vi "PositionReceiverAngleAttacker.vi"(6 "AnguloGol":dbl, 8 "error in (no error)":errorcluster, 9 "atacando contra":bool, 10 "Game":refnum<class "Game.lvclass">, 11 "PositionToReceivePassSkill in":refnum<class "PositionToReceivePassSkill.lvclass">) -> (0 "error out":errorcluster, 1 "AttackerPositive?":bool, 2 "theta final":dbl, 3 "PositionToReceivePassSkill out":refnum<class "PositionToReceivePassSkill.lvclass">, 4 "YdoAttacker 2":dbl, 5 "XdoAttacker 2":dbl)   [LabVIEW 2023, in "PositionToReceivePassSkill.lvclass"]
uses:
  PositionToReceivePassSkill.lvclass
  Game_class/Game.lvclass
  Game_class/Game.lvclass/Game.ctl
  Team_class/Team.lvclass/Team.ctl
  Object_class/Object.lvclass/Object.ctl
  Robot_class/Robot.lvclass/Robot.ctl
  Object_class/Read x.vi
  Object_class/Write x.vi
  Object_class/Read y.vi
  Robot_class/Read id.vi
  Game_class/Read OffensiveTeam.vi
  Game_class/Read EnemyRef.vi
  Game_class/Read FieldRef.vi
  Game_class/Read DefensiveTeam.vi
  Game_class/Read KeeperTeam.vi
  Game_class/Read BallRef.vi
  Team_class/Read RobotRef.vi
  Ball_class/Ball.lvclass
  Ally_class/Ally.lvclass
  Enemy_class/Enemy.lvclass
  Robot_class/Robot.lvclass
  Field_class/Field.lvclass
panel:
  in  "valor de theta 3":dbl
  in  "tamanho do intervalo 3":dbl
  in  "inicio do intervalo 3":dbl
  in  "fim do intervalo 3":dbl
  in  "Contador 4":dbl
  in  "Array 3":dbl[](array[numeric])=[0.0, 0.0, 0.0, 0.0, 0.0, 0.0]
  in  "valor de theta 2":dbl
  in  "tamanho do intervalo 2":dbl
  in  "inicio do intervalo 2":dbl
  in  "fim do intervalo 2":dbl
  in  "Contador 3":dbl
  in  "Array 2":dbl[](array[numeric])=[0.0, 0.0, 0.0, 0.0, 0.0, 0.0]
  in  "RobôsParaAnalisar":dbl[][](array[numeric])=[[99999.0, 99999.0], [99999.0, 99999.0], [99999.0, 99999.0], [99999.0, 99999.0], [99999.0, 99999.0], [99999.0, 99999.0], [99999.0, 99999.0]]
  in  "Contador":dbl
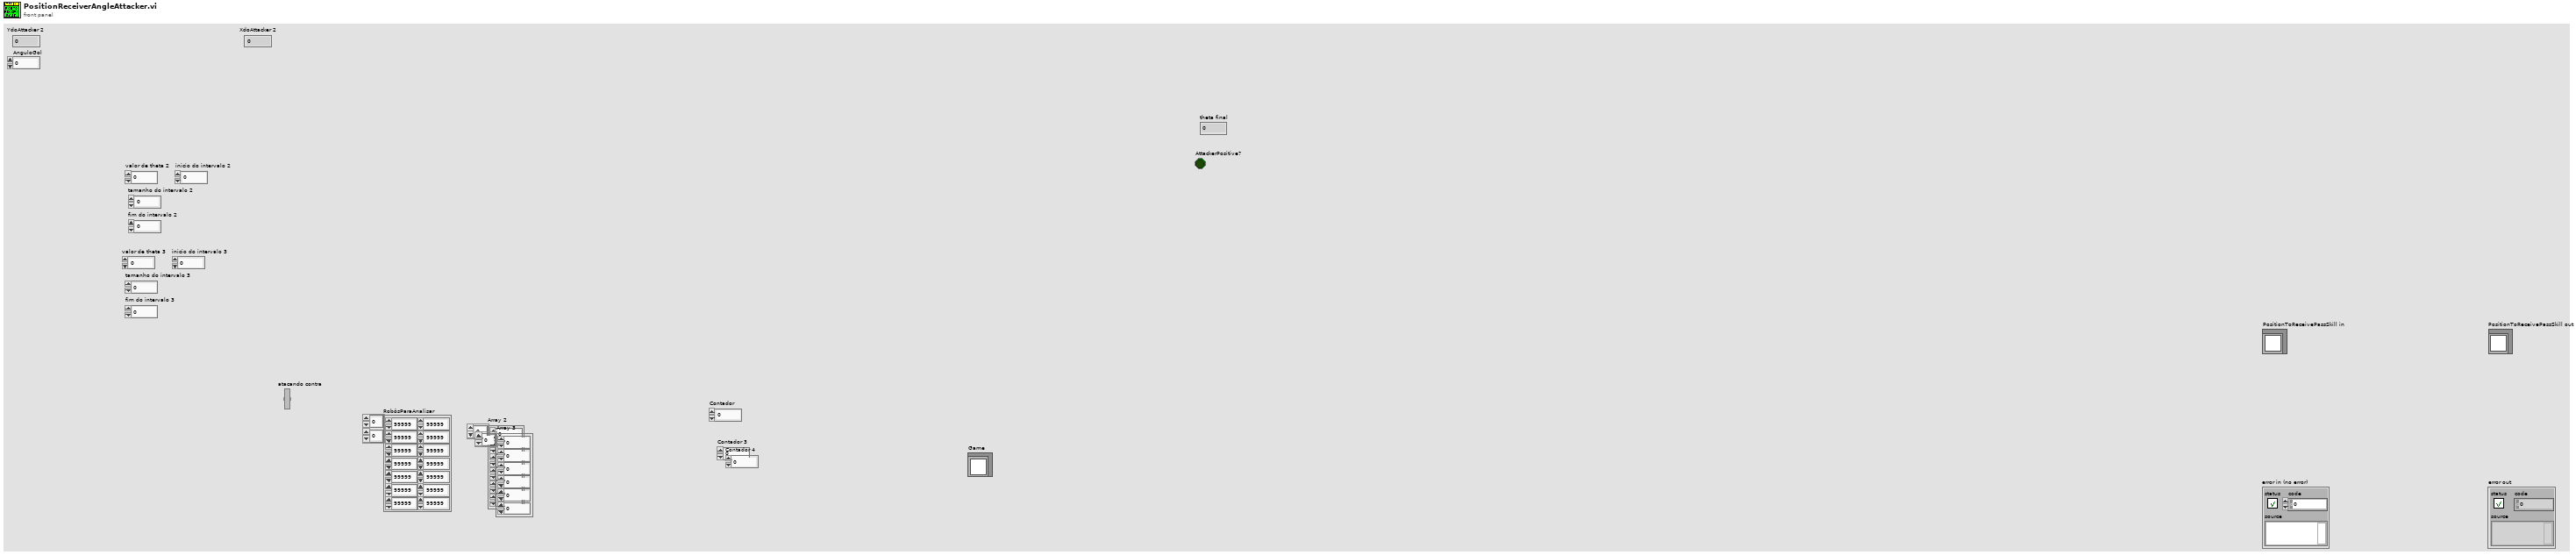
[diagram p1: front panel]
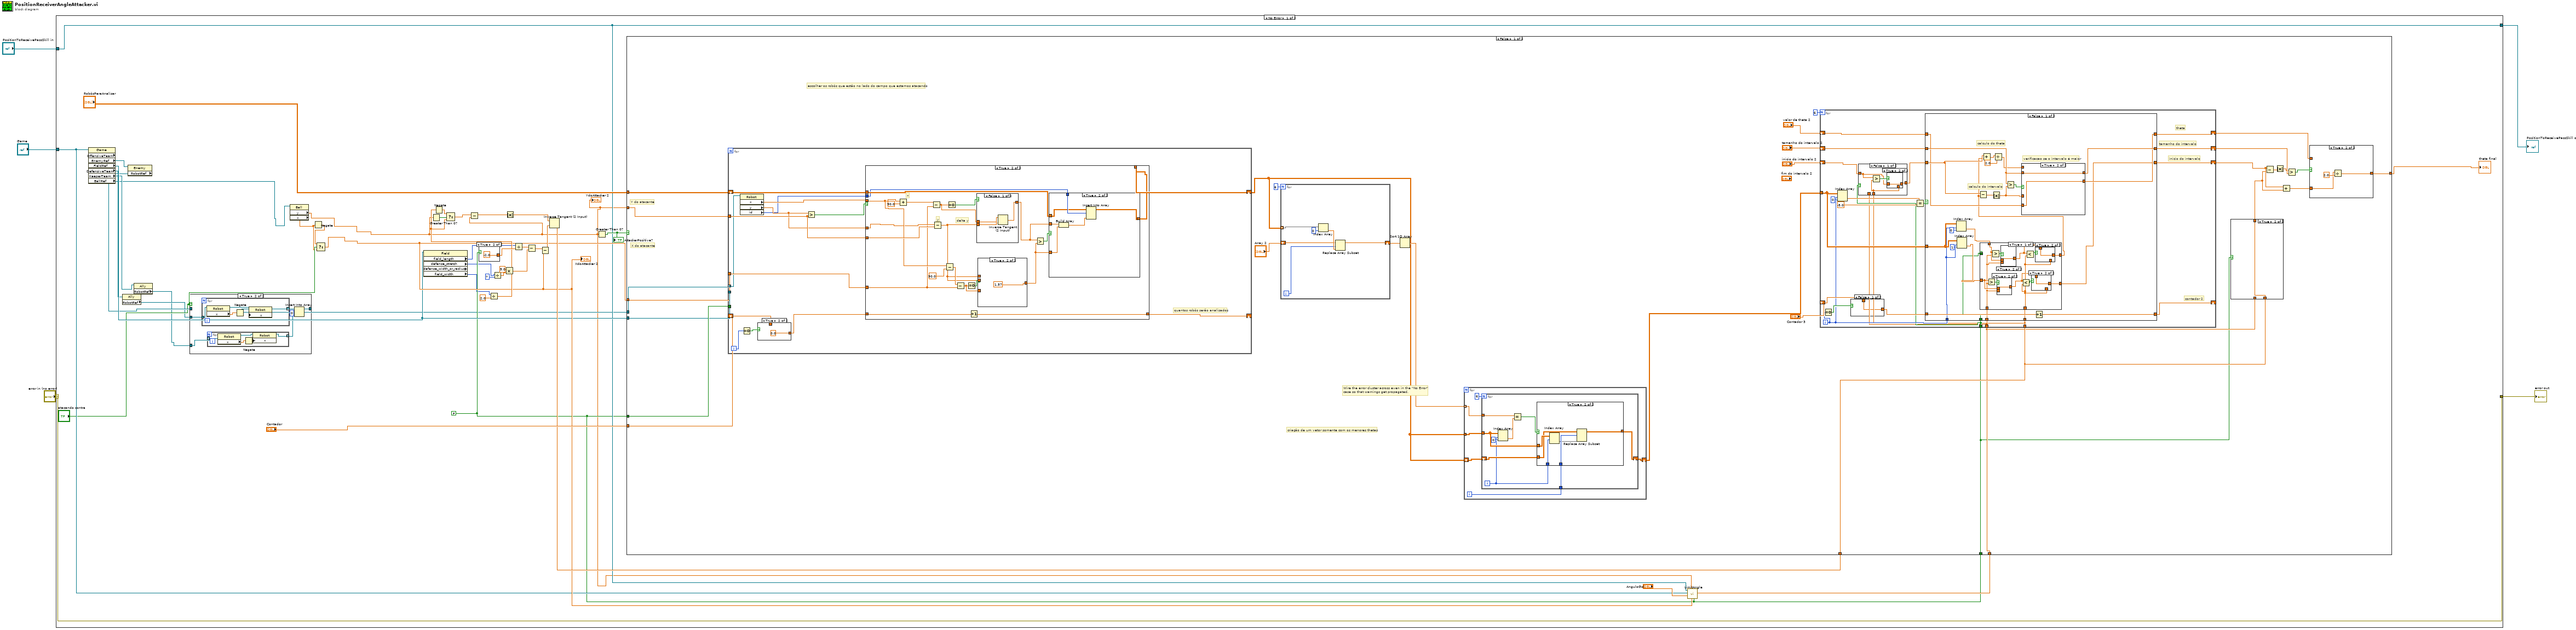
[diagram p0: block diagram]
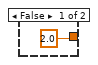
[diagram p3: hidden frame]
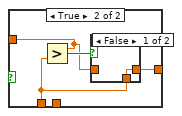
[diagram p8: hidden frame]
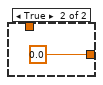
[diagram p10: hidden frame]
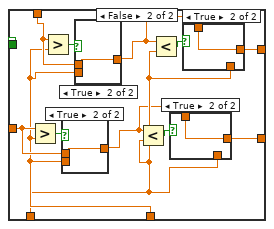
[diagram p15: hidden frame]
diagram:
  n1 = case shown="No Error" "error in (no error)" {
    selector: "error in (no error)" -> [w48 w537]
    tunnel: [w48 w537] -> w4
    tunnel: [w25 w536] -> w2
    tunnel: "PositionToReceivePassSkill in" -> [w25 w536]
    tunnel: "Game" -> [w26 _]
    frame No Error {
      w20 = FALSE ("atacando contra")
      # "Wire the error cluster across even in the \"No Error\"\ncase so that warnings get propagated."
      n2 = property class="Game" props=["OffensiveTeam", "EnemyRef", "FieldRef", "DefensiveTeam", "KeeperTeam", "BallRef"](reference=w26) -> ("EnemyRef"=w29:refnum<class "Enemy.lvclass">, "FieldRef"=w28:refnum<class "Field.lvclass">, "DefensiveTeam"=w15:refnum<class "Ally.lvclass">, "KeeperTeam"=w13:refnum<class "Ally.lvclass">, "BallRef"=w11:refnum<class "Ball.lvclass">)  [unwired: 1 in, 3 out]
      n3 = property class="Ally"(reference=w15) -> ("RobotRef"=w14:refnum<class "Robot.lvclass">[])  [unwired: 1 in, 2 out]
      n4 = property class="Enemy"(reference=w29) -> ("RobotRef"=w18:refnum<class "Robot.lvclass">[])  [unwired: 1 in, 2 out]
      n5 = property class="Ally"(reference=w13) -> ("RobotRef"=w12:refnum<class "Robot.lvclass">[])  [unwired: 1 in, 2 out]
      n6 = case shown="True" "atacando contra" {
        tunnel: [w49 w50] -> w19
        tunnel: w18 -> [w49 _]
        tunnel: w14 -> [_ w55]
        tunnel: w12 -> [_ w54]
        frame False {
        }
        frame True {
          n7 = for {
            tunnel: [w63] -> w53 mode=indexing
            tunnel: w55 -> [w61] mode=indexing
            n8 = property class="Robot"(reference=w61) -> (reference out=w62:refnum<class "Robot.lvclass">, "x"=w65:dbl)  [unwired: 1 in, 1 out]
            n9 = Negate(x=w65) -> (-x=w64:dbl)
            n10 = property class="Robot"(reference=w62, "x"=w64) -> (reference out=w63:refnum<class "Robot.lvclass">)  [unwired: 1 in, 1 out]
          }
          n11 = for {
            tunnel: w54 -> [w60] mode=indexing
            tunnel: [w56] -> w52 mode=indexing
            n12 = property class="Robot"(reference=w60) -> (reference out=w57:refnum<class "Robot.lvclass">, "x"=w59:dbl)  [unwired: 1 in, 1 out]
            n13 = Negate(x=w59) -> (-x=w58:dbl)
            n14 = property class="Robot"(reference=w57, "x"=w58) -> (reference out=w56:refnum<class "Robot.lvclass">)  [unwired: 1 in, 1 out]
          }
          n15 = Insert Into Array(array=w53, index=0, new element=w52) -> (w50:refnum<class "Robot.lvclass">[])
        }
      }
      n16 = property class="Ball"(reference=w11) -> ("y"=w9:dbl, "x"=w8:dbl)  [unwired: 1 in, 2 out]
      "YdoAttacker 2" <- w9
      n17 = Negate(x=w8) -> (-x=w10:dbl)
      n18 = Select(t=w10, s="atacando contra", f=w8) -> (s? t:f=w34:dbl)
      "XdoAttacker 2" <- w34
      n19 = property class="Field" props=["field_length", "defense_stretch", "defense_width_or_radius", "field_width"](reference=w28) -> ("field_length"=w27:i32, "defense_stretch"=w7:i32, "field_width"=w6:i32)  [unwired: 1 in, 3 out]
      n20 = Greater Than 0?(x=w9) -> (x > 0?=w44:bool)
      n21 = case shown="True" w20 {
        tunnel: [2.0 ("y") -2.0 ("y")] -> w42
        frame False {
        }
        frame True {
        }
      }
      n22 = Divide(x=w6, y=2.0) -> (x/y=w40:dbl)
      n23 = Negate(x=w40) -> (-x=w43:dbl)
      n24 = Select(t=w43, s=w44, f=w40) -> (s? t:f=w36:dbl)
      n25 = Subtract(x=w36, y=w9) -> (x-y=w33:dbl)
      n26 = Divide(x=w7, y=7) -> (x/y=w23:dbl)
      n27 = Multiply(x=5.0, y=w23) -> (x*y=w21:dbl)
      n28 = Absolute Value(x=w33) -> (abs(x)=w32:dbl)
      n29 = Divide(x=w27, y=w42) -> (x/y=w31:dbl)
      n30 = Subtract(x=w31, y=w21) -> (x-y=w30:dbl)
      n31 = Subtract(x=w30, y=w34) -> (x-y=w35:dbl)
      n32 = Inverse Tangent (2 Input)(1:w35, 2:w32) -> (0:w39:dbl)
      n33 = Greater Than 0?(x=w9) -> (x > 0?=w45:bool)
      "AttackerPositive?" <- w45
      n34 = call-dynamic "LimitAngle.vi"("atacando contra"=w20, "XdoAttacker"=w34, "YdoAttacker"=w9, "AnguloGol"="AnguloGol", "Game"=w26, "PositionToReceivePassSkill in"=w25) -> ("Angulo Limite"=w37:dbl)  [unwired: 3 in, 2 out]
      n35 = case shown="False" w45 {
        tunnel: w19 -> [w97 w330]
        tunnel: w20 -> [w96 w329]
        tunnel: "Contador" -> [w95 w328]
        tunnel: "RobôsParaAnalisar" -> [w94 w327]
        tunnel: w28 -> [w93 w326]
        tunnel: [w79 w312] -> w16
        tunnel: w9 -> [w73 w306]
        tunnel: w34 -> [w72 w305]
        tunnel: w39 -> [w70 w301]
        tunnel: w20 -> [w68 w304]
        tunnel: w37 -> [w69 w303]
        frame False {
          # "X do atacante"
          # "Y do atacante"
          # "criação de um vetor somente com os menores thetas"
          # "escolher os robôs que estão no lado do campo que estamos atacando"
          n36 = for {
            tunnel: w97 -> [w241] mode=indexing
            tunnel: w96 -> [_]
            shift-right: [w245] -> w83
            shift-left: w94 -> [w251]
            shift-right: [w246] -> _
            shift-left: w95 -> [w248]
            tunnel: w93 -> [_]
            tunnel: w73 -> [w243]
            tunnel: w72 -> [w242]
            i -> [w249]
            # "quantos robôs serão analisados"
            n37 = property class="Robot"(reference=w241) -> ("x"=w240:dbl, "y"=w239:dbl, "id"=w238:i32)  [unwired: 1 in, 2 out]
            n38 = Equal To 0?(x=w249) -> (x = 0?=w250:bool)
            n39 = case shown="True" w250 {
              tunnel: w248 -> [w252 _]
              tunnel: [w252 0.0] -> w247
              frame False {
              }
              frame True {
              }
            }
            n40 = Greater?(x=w239, y=w243) -> (0:w244:bool)
            n41 = case shown="True" w244 {
              tunnel: w251 -> [w258 w278]
              tunnel: w238 -> [w257 w277]
              tunnel: w240 -> [_ w268]
              tunnel: w239 -> [_ w267]
              tunnel: w247 -> [w259 w279]
              tunnel: [w259 w280] -> w246
              tunnel: [w254 w276] -> w245
              tunnel: w243 -> [_ w269]
              tunnel: w242 -> [_ w265]
              frame False {
                w256 = -5.0 ("element")
                n42 = Build Array(w256, w256) -> (w255:dbl[])
                n43 = Insert Into Array(array=w258, index (row)=w257, new element=w255) -> (w254:dbl[][])  [unwired: 1 in]
              }
              frame True {
                # "delta y"
                # "y"
                # "x"
                n44 = Add(x=w268, y=90.0) -> (x+y=w266:dbl)
                n45 = Subtract(x=w266, y=w265) -> (x-y=w263:dbl)
                n46 = Subtract(x=w267, y=w269) -> (x-y=w260:dbl)
                n47 = Subtract(x=w268, y=90.0) -> (x-y=w273:dbl)
                n48 = Equal To 0?(x=w263) -> (x = 0?=w264:bool)
                n49 = Subtract(x=w273, y=w265) -> (x-y=w261:dbl)
                n50 = Equal To 0?(x=w261) -> (x = 0?=w262:bool)
                n51 = Increment(x=w279) -> (x+1=w280:dbl)
                n52 = case shown="False" w264 {
                  tunnel: [w298 1.57] -> w271
                  tunnel: w260 -> [w299 _]
                  tunnel: w263 -> [w297 _]
                  frame False {
                    n53 = Inverse Tangent (2 Input)(1:w297, 2:w299) -> (0:w298:dbl)
                  }
                  frame True {
                  }
                }
                n54 = case shown="True" w262 {
                  tunnel: [w283 1.57] -> w270
                  tunnel: w260 -> [_ _]
                  tunnel: w261 -> [w282 _]
                  tunnel: w260 -> [w281 _]
                  frame False {
                    n55 = Inverse Tangent (2 Input)(1:w282, 2:w281) -> (0:w283:dbl)
                  }
                  frame True {
                  }
                }
                n56 = Greater?(x=w271, y=w270) -> (0:w272:bool)
                n57 = case shown="True" w272 {
                  tunnel: w278 -> [w287 w293]
                  tunnel: w277 -> [w289 w296]
                  tunnel: w271 -> [w286 w294]
                  tunnel: w270 -> [w288 w292]
                  tunnel: [w285 w291] -> w276
                  frame False {
                    n58 = Build Array(w288, w286) -> (w290:dbl[])
                    n59 = Insert Into Array(array=w287, index (row)=w289, new element=w290) -> (w285:dbl[][])  [unwired: 1 in]
                  }
                  frame True {
                    n60 = Build Array(w294, w292) -> (w295:dbl[])
                    n61 = Insert Into Array(array=w293, index (row)=w296, new element=w295) -> (w291:dbl[][])  [unwired: 1 in]
                  }
                }
              }
            }
          }
          n62 = for {
            N: 6 -> [_]
            tunnel: w83 -> [w131] mode=indexing
            shift-right: [w126] -> w85
            shift-left: "Array 2" -> [w127]
            i -> [w128]
            n63 = Index Array(array=w131, index=0) -> (element=w129:dbl)
            n64 = Replace Array Subset(array=w127, new element=w129, index=w128) -> (w126:dbl[])
          }
          n65 = Sort 1D Array(array=w85) -> (sorted array=w84:dbl[])
          n66 = for {
            tunnel: w84 -> [w106] mode=indexing
            tunnel: w83 -> [w108]
            shift-right: [w104] -> w82
            shift-left: w83 -> [w107]
            i -> [w105]
            n67 = for {
              N: 6 -> [_]
              tunnel: w108 -> [w114]
              shift-right: [w110] -> w104
              shift-left: w107 -> [w113]
              tunnel: w106 -> [w116]
              tunnel: w105 -> [w111]
              i -> [w112]
              n68 = Index Array(array=w114, index (row)=w112, index (col)=0 ("disabled index (col)")) -> (element=w117:dbl)
              n69 = Equal?(x=w116, y=w117) -> (x = y?=w115:bool)
              n70 = case shown="True" w115 {
                tunnel: w114 -> [_ w125]
                tunnel: w113 -> [w119 w121]
                tunnel: w112 -> [_ w124]
                tunnel: w111 -> [_ w123]
                tunnel: [w119 w120] -> w110
                frame False {
                }
                frame True {
                  n71 = Index Array(array=w125, index (row)=w124) -> (element=w122:dbl[])  [unwired: 1 in]
                  n72 = Replace Array Subset(array=w121, new element=w122, index (row)=w123) -> (w120:dbl[][])  [unwired: 1 in]
                }
              }
            }
          }
          n73 = for {
            N: 6 -> [_]
            tunnel: w82 -> [w138]
            shift-right: [w146] -> w78
            shift-left: "valor de theta 2" -> [w147]
            shift-right: [w144] -> w81
            shift-left: "tamanho do intervalo 2" -> [w145]
            shift-right: [w143] -> w75
            shift-left: "inicio do intervalo 2" -> [w135]
            shift-right: [w139] -> _
            shift-left: "Contador 3" -> [w141]
            tunnel: w69 -> [w133]
            tunnel: w70 -> [w132]
            tunnel: w68 -> [w136]
            i -> [w137]
            # "contador 2"
            # "inicio do intervalo"
            # "tamanho do intervalo"
            # "theta"
            n74 = Equal To 0?(x=w137) -> (x = 0?=w142:bool)
            n75 = Index Array(array=w138, index (row)=w137, index (col)=0 ("disabled index (col)")) -> (element=w149:dbl)
            n76 = case shown="False" w142 {
              tunnel: w141 -> [w164 _]
              tunnel: [w164 0.0] -> w140
              frame False {
              }
              frame True {
              }
            }
            n77 = case shown="False" w136 {
              tunnel: w133 -> [_ w158]
              tunnel: w135 -> [w154 w159]
              tunnel: [w152 w160] -> w134
              tunnel: w132 -> [w153 _]
              frame False {
                n78 = Greater?(x=w154, y=w153) -> (0:w155:bool)
                n79 = case shown="True" w155 {
                  tunnel: [w156 w157] -> w152
                  tunnel: w154 -> [_ w157]
                  tunnel: w153 -> [w156 _]
                  frame False {
                  }
                  frame True {
                  }
                }
              }
              frame True {
                n80 = Greater?(x=w159, y=w158) -> (0:w161:bool)
                n81 = case shown="False" w161 {
                  tunnel: [w162 w163] -> w160
                  tunnel: w159 -> [_ w163]
                  tunnel: w158 -> [w162 _]
                  frame False {
                  }
                  frame True {
                  }
                }
              }
            }
            n82 = Equal?(x=w149, y=-5.0) -> (x = y?=w150:bool)
            n83 = case shown="False" w150 {
              tunnel: w147 -> [w173 w237]
              tunnel: [w174 w237] -> w146
              tunnel: w145 -> [w178 w236]
              tunnel: [w177 w236] -> w144
              tunnel: w134 -> [w189 w235]
              tunnel: [w172 w235] -> w143
              tunnel: w140 -> [w187 w234]
              tunnel: [w188 w234] -> w139
              tunnel: w138 -> [w186 _]
              tunnel: w137 -> [w185 _]
              tunnel: w133 -> [w169 _]
              tunnel: w132 -> [w170 _]
              tunnel: w136 -> [w166 _]
              frame False {
                # "calculo do theta"
                # "calculo do intervalo"
                # "verificacao se o intervalo é maior"
                n84 = Index Array(array=w186, index (row)=w185, index (col)=0 ("disabled index (col)")) -> (element=w168:dbl)
                n85 = Index Array(array=w186, index (row)=w185, index (col)=1 ("disabled index (col)")) -> (element=w167:dbl)
                n86 = case shown="True" w166 {
                  tunnel: w169 -> [w193 w211]
                  tunnel: w168 -> [w200 w220]
                  tunnel: w170 -> [w192 w212]
                  tunnel: [w198 w218] -> w171
                  tunnel: w167 -> [w194 w214]
                  tunnel: [w191 w213] -> w172
                  tunnel: w166 -> [_ _]
                  frame True {
                    n87 = Greater?(x=w194, y=w193) -> (0:w196:bool)
                    n88 = Greater?(x=w200, y=w193) -> (0:w201:bool)
                    n89 = case shown="True" w196 {
                      tunnel: [w204 w205] -> w190
                      tunnel: w194 -> [_ w205]
                      tunnel: w193 -> [w204 _]
                      frame False {
                      }
                      frame True {
                      }
                    }
                    n90 = case shown="True" w201 {
                      tunnel: [w208 w209] -> w197
                      tunnel: w200 -> [_ w209]
                      tunnel: w193 -> [w208 _]
                      frame False {
                      }
                      frame True {
                      }
                    }
                    n91 = Less?(x=w190, y=w192) -> (x < y?=w195:bool)
                    n92 = Less?(x=w197, y=w192) -> (x < y?=w199:bool)
                    n93 = case shown="True" w195 {
                      tunnel: [w202 w203] -> w191
                      tunnel: w190 -> [_ w203]
                      tunnel: w192 -> [w202 _]
                      frame False {
                      }
                      frame True {
                      }
                    }
                    n94 = case shown="True" w199 {
                      tunnel: [w206 w207] -> w198
                      tunnel: w197 -> [_ w207]
                      tunnel: w192 -> [w206 _]
                      frame False {
                      }
                      frame True {
                      }
                    }
                  }
                  frame False {
                    n95 = Greater?(x=w214, y=w212) -> (0:w216:bool)
                    n96 = Greater?(x=w220, y=w212) -> (0:w221:bool)
                    n97 = case shown="True" w216 {
                      tunnel: [w224 w225] -> w210
                      tunnel: w214 -> [_ w225]
                      tunnel: w212 -> [w224 _]
                      frame False {
                      }
                      frame True {
                      }
                    }
                    n98 = case shown="True" w221 {
                      tunnel: [w228 w229] -> w217
                      tunnel: w220 -> [_ w229]
                      tunnel: w212 -> [w228 _]
                      frame False {
                      }
                      frame True {
                      }
                    }
                    n99 = Less?(x=w210, y=w211) -> (x < y?=w215:bool)
                    n100 = Less?(x=w217, y=w211) -> (x < y?=w219:bool)
                    n101 = case shown="True" w215 {
                      tunnel: [w222 w223] -> w213
                      tunnel: w210 -> [_ w223]
                      tunnel: w211 -> [w222 _]
                      frame False {
                      }
                      frame True {
                      }
                    }
                    n102 = case shown="True" w219 {
                      tunnel: [w226 w227] -> w218
                      tunnel: w217 -> [_ w227]
                      tunnel: w211 -> [w226 _]
                      frame False {
                      }
                      frame True {
                      }
                    }
                  }
                }
                n103 = Subtract(x=w189, y=w171) -> (x-y=w182:dbl)
                n104 = Add(x=w189, y=w171) -> (x+y=w181:dbl)
                n105 = Absolute Value(x=w182) -> (abs(x)=w176:dbl)
                n106 = Divide(x=w181, y=2.0) -> (x/y=w175:dbl)
                n107 = Greater?(x=w178, y=w176) -> (0:w179:bool)
                n108 = case shown="True" w179 {
                  tunnel: w178 -> [_ w233]
                  tunnel: [w231 w233] -> w177
                  tunnel: w176 -> [w231 _]
                  tunnel: w173 -> [_ w232]
                  tunnel: w175 -> [w230 _]
                  tunnel: [w230 w232] -> w174
                  frame False {
                  }
                  frame True {
                  }
                }
                n109 = Increment(x=w187) -> (x+1=w188:dbl)
              }
              frame True {
              }
            }
          }
          n110 = case shown="True" w68 {
            tunnel: w69 -> [w98 _]
            tunnel: [w98 w99] -> w71
            tunnel: w70 -> [_ w99]
            frame False {
            }
            frame True {
            }
          }
          n111 = Subtract(x=w75, y=w71) -> (x-y=w77:dbl)
          n112 = Absolute Value(x=w77) -> (abs(x)=w76:dbl)
          n113 = Add(x=w75, y=w71) -> (x+y=w74:dbl)
          n114 = Greater?(x=w76, y=w81) -> (0:w80:bool)
          n115 = case shown="True" w80 {
            tunnel: [w100 w102] -> w79
            tunnel: w78 -> [w100 _]
            tunnel: w74 -> [_ w101]
            frame False {
            }
            frame True {
              n116 = Divide(x=w101, y=2.0) -> (x/y=w102:dbl)
            }
          }
        }
        frame True {
          # "X do atacante"
          # "Y do atacante"
          # "criação de um vetor somente com os menores thetas"
          # "escolher os robôs que estão no lado do campo que estamos atacando"
          n117 = for {
            tunnel: w330 -> [w474] mode=indexing
            tunnel: w329 -> [_]
            shift-right: [w478] -> w316
            shift-left: w327 -> [w484]
            shift-right: [w479] -> _
            shift-left: w328 -> [w481]
            tunnel: w326 -> [_]
            tunnel: w306 -> [w476]
            tunnel: w305 -> [w475]
            i -> [w482]
            # "quantos robôs serão analisados"
            n118 = Equal To 0?(x=w482) -> (x = 0?=w483:bool)
            n119 = property class="Robot"(reference=w474) -> ("x"=w473:dbl, "y"=w471:dbl, "id"=w472:i32)  [unwired: 1 in, 2 out]
            n120 = case shown="True" w483 {
              tunnel: w481 -> [w485 _]
              tunnel: [w485 0.0] -> w480
              frame False {
              }
              frame True {
              }
            }
            n121 = Less?(x=w471, y=w476) -> (x < y?=w477:bool)
            n122 = case shown="True" w477 {
              tunnel: w484 -> [w491 w511]
              tunnel: w472 -> [w487 w510]
              tunnel: w473 -> [_ w493]
              tunnel: w480 -> [w492 w512]
              tunnel: [w492 w513] -> w479
              tunnel: [w488 w509] -> w478
              tunnel: w476 -> [_ w502]
              tunnel: w475 -> [_ w500]
              tunnel: w471 -> [_ w494]
              frame False {
                w490 = -5.0 ("element")
                n123 = Build Array(w490, w490) -> (w489:dbl[])
                n124 = Insert Into Array(array=w491, index (row)=w487, new element=w489) -> (w488:dbl[][])  [unwired: 1 in]
              }
              frame True {
                # "delta y"
                # "y"
                # "x"
                n125 = Add(x=w493, y=90.0) -> (x+y=w501:dbl)
                n126 = Subtract(x=w501, y=w500) -> (x-y=w498:dbl)
                n127 = Subtract(x=w494, y=w502) -> (x-y=w495:dbl)
                n128 = Subtract(x=w493, y=90.0) -> (x-y=w506:dbl)
                n129 = Equal To 0?(x=w498) -> (x = 0?=w499:bool)
                n130 = Subtract(x=w506, y=w500) -> (x-y=w496:dbl)
                n131 = Equal To 0?(x=w496) -> (x = 0?=w497:bool)
                n132 = Increment(x=w512) -> (x+1=w513:dbl)
                n133 = case shown="True" w499 {
                  tunnel: [w534 1.57] -> w504
                  tunnel: w495 -> [w532 _]
                  tunnel: w498 -> [w533 _]
                  frame False {
                    n134 = Absolute Value(x=w532) -> (abs(x)=w531:dbl)
                    n135 = Inverse Tangent (2 Input)(1:w533, 2:w531) -> (0:w534:dbl)
                  }
                  frame True {
                  }
                }
                n136 = case shown="True" w497 {
                  tunnel: [w517 1.57] -> w503
                  tunnel: w495 -> [_ _]
                  tunnel: w496 -> [w516 _]
                  tunnel: w495 -> [w514 _]
                  frame False {
                    n137 = Absolute Value(x=w514) -> (abs(x)=w515:dbl)
                    n138 = Inverse Tangent (2 Input)(1:w516, 2:w515) -> (0:w517:dbl)
                  }
                  frame True {
                  }
                }
                n139 = Greater?(x=w504, y=w503) -> (0:w505:bool)
                n140 = case shown="False" w505 {
                  tunnel: w511 -> [w522 w528]
                  tunnel: w510 -> [w519 w525]
                  tunnel: w504 -> [w521 w529]
                  tunnel: w503 -> [w523 w527]
                  tunnel: [w520 w526] -> w509
                  frame False {
                    n141 = Build Array(w523, w521) -> (w524:dbl[])
                    n142 = Insert Into Array(array=w522, index (row)=w519, new element=w524) -> (w520:dbl[][])  [unwired: 1 in]
                  }
                  frame True {
                    n143 = Build Array(w529, w527) -> (w530:dbl[])
                    n144 = Insert Into Array(array=w528, index (row)=w525, new element=w530) -> (w526:dbl[][])  [unwired: 1 in]
                  }
                }
              }
            }
          }
          n145 = for {
            N: 6 -> [_]
            tunnel: w316 -> [w364] mode=indexing
            shift-right: [w359] -> w318
            shift-left: "Array 3" -> [w360]
            i -> [w361]
            n146 = Index Array(array=w364, index=0) -> (element=w362:dbl)
            n147 = Replace Array Subset(array=w360, new element=w362, index=w361) -> (w359:dbl[])
          }
          n148 = Sort 1D Array(array=w318) -> (sorted array=w317:dbl[])
          n149 = for {
            tunnel: w317 -> [w339] mode=indexing
            tunnel: w316 -> [w341]
            shift-right: [w337] -> w315
            shift-left: w316 -> [w340]
            i -> [w338]
            n150 = for {
              N: 6 -> [_]
              tunnel: w341 -> [w347]
              shift-right: [w343] -> w337
              shift-left: w340 -> [w346]
              tunnel: w339 -> [w349]
              tunnel: w338 -> [w344]
              i -> [w345]
              n151 = Index Array(array=w347, index (row)=w345, index (col)=0 ("disabled index (col)")) -> (element=w350:dbl)
              n152 = Equal?(x=w349, y=w350) -> (x = y?=w348:bool)
              n153 = case shown="False" w348 {
                tunnel: w347 -> [_ w358]
                tunnel: w346 -> [w352 w354]
                tunnel: w345 -> [_ w357]
                tunnel: w344 -> [_ w356]
                tunnel: [w352 w353] -> w343
                frame False {
                }
                frame True {
                  n154 = Index Array(array=w358, index (row)=w357) -> (element=w355:dbl[])  [unwired: 1 in]
                  n155 = Replace Array Subset(array=w354, new element=w355, index (row)=w356) -> (w353:dbl[][])  [unwired: 1 in]
                }
              }
            }
          }
          n156 = for {
            N: 6 -> [_]
            tunnel: w315 -> [w371]
            shift-right: [w379] -> w311
            shift-left: "valor de theta 3" -> [w380]
            shift-right: [w377] -> w314
            shift-left: "tamanho do intervalo 3" -> [w378]
            shift-right: [w376] -> w308
            shift-left: "inicio do intervalo 3" -> [w367]
            shift-right: [w372] -> _
            shift-left: "Contador 4" -> [w374]
            tunnel: w304 -> [w369]
            tunnel: w303 -> [w368]
            tunnel: w301 -> [w365]
            i -> [w370]
            # "contador 2"
            # "inicio do intervalo"
            # "tamanho do intervalo"
            # "theta"
            n157 = Equal To 0?(x=w370) -> (x = 0?=w375:bool)
            n158 = Index Array(array=w371, index (row)=w370, index (col)=1 ("disabled index (col)")) -> (element=w382:dbl)
            n159 = case shown="False" w375 {
              tunnel: w374 -> [w397 _]
              tunnel: [w397 0.0] -> w373
              frame False {
              }
              frame True {
              }
            }
            n160 = case shown="False" w369 {
              tunnel: w368 -> [_ w391]
              tunnel: w367 -> [w387 w392]
              tunnel: [w385 w393] -> w366
              tunnel: w365 -> [w386 _]
              frame False {
                n161 = Greater?(x=w387, y=w386) -> (0:w388:bool)
                n162 = case shown="True" w388 {
                  tunnel: [w389 w390] -> w385
                  tunnel: w387 -> [_ w390]
                  tunnel: w386 -> [w389 _]
                  frame False {
                  }
                  frame True {
                  }
                }
              }
              frame True {
                n163 = Greater?(x=w392, y=w391) -> (0:w394:bool)
                n164 = case shown="False" w394 {
                  tunnel: [w395 w396] -> w393
                  tunnel: w392 -> [_ w396]
                  tunnel: w391 -> [w395 _]
                  frame False {
                  }
                  frame True {
                  }
                }
              }
            }
            n165 = Equal?(x=w382, y=-5.0) -> (x = y?=w383:bool)
            n166 = case shown="False" w383 {
              tunnel: w380 -> [w407 w470]
              tunnel: [w408 w470] -> w379
              tunnel: w378 -> [w412 w469]
              tunnel: [w411 w469] -> w377
              tunnel: [w401 w467] -> w376
              tunnel: w373 -> [w421 w468]
              tunnel: [w422 w468] -> w372
              tunnel: w371 -> [w420 _]
              tunnel: w370 -> [w419 _]
              tunnel: w369 -> [w406 _]
              tunnel: w368 -> [w405 _]
              tunnel: w365 -> [w404 _]
              tunnel: w366 -> [w400 w467]
              frame False {
                # "calculo do theta"
                # "calculo do intervalo"
                # "verificacao se o intervalo é maior"
                n167 = Index Array(array=w420, index (row)=w419, index (col)=1 ("disabled index (col)")) -> (element=w399:dbl)
                n168 = Index Array(array=w420, index (row)=w419, index (col)=0 ("disabled index (col)")) -> (element=w402:dbl)
                n169 = case shown="False" w406 {
                  tunnel: w405 -> [w426 w444]
                  tunnel: w399 -> [w433 w453]
                  tunnel: w404 -> [w425 w445]
                  tunnel: [w431 w451] -> w403
                  tunnel: w402 -> [w427 w447]
                  tunnel: [w424 w446] -> w401
                  frame True {
                    n170 = Greater?(x=w427, y=w426) -> (0:w429:bool)
                    n171 = Greater?(x=w433, y=w426) -> (0:w434:bool)
                    n172 = case shown="True" w429 {
                      tunnel: [w437 w438] -> w423
                      tunnel: w427 -> [_ w438]
                      tunnel: w426 -> [w437 _]
                      frame False {
                      }
                      frame True {
                      }
                    }
                    n173 = case shown="True" w434 {
                      tunnel: [w441 w442] -> w430
                      tunnel: w433 -> [_ w442]
                      tunnel: w426 -> [w441 _]
                      frame False {
                      }
                      frame True {
                      }
                    }
                    n174 = Less?(x=w423, y=w425) -> (x < y?=w428:bool)
                    n175 = Less?(x=w430, y=w425) -> (x < y?=w432:bool)
                    n176 = case shown="False" w428 {
                      tunnel: [w435 w436] -> w424
                      tunnel: w423 -> [_ w436]
                      tunnel: w425 -> [w435 _]
                      frame False {
                      }
                      frame True {
                      }
                    }
                    n177 = case shown="True" w432 {
                      tunnel: [w439 w440] -> w431
                      tunnel: w430 -> [_ w440]
                      tunnel: w425 -> [w439 _]
                      frame False {
                      }
                      frame True {
                      }
                    }
                  }
                  frame False {
                    n178 = Greater?(x=w447, y=w445) -> (0:w449:bool)
                    n179 = Greater?(x=w453, y=w445) -> (0:w454:bool)
                    n180 = case shown="True" w449 {
                      tunnel: [w457 w458] -> w443
                      tunnel: w447 -> [_ w458]
                      tunnel: w445 -> [w457 _]
                      frame False {
                      }
                      frame True {
                      }
                    }
                    n181 = case shown="True" w454 {
                      tunnel: [w461 w462] -> w450
                      tunnel: w453 -> [_ w462]
                      tunnel: w445 -> [w461 _]
                      frame False {
                      }
                      frame True {
                      }
                    }
                    n182 = Less?(x=w443, y=w444) -> (x < y?=w448:bool)
                    n183 = Less?(x=w450, y=w444) -> (x < y?=w452:bool)
                    n184 = case shown="True" w448 {
                      tunnel: [w455 w456] -> w446
                      tunnel: w443 -> [_ w456]
                      tunnel: w444 -> [w455 _]
                      frame False {
                      }
                      frame True {
                      }
                    }
                    n185 = case shown="True" w452 {
                      tunnel: [w459 w460] -> w451
                      tunnel: w450 -> [_ w460]
                      tunnel: w444 -> [w459 _]
                      frame False {
                      }
                      frame True {
                      }
                    }
                  }
                }
                n186 = Subtract(x=w400, y=w403) -> (x-y=w416:dbl)
                n187 = Add(x=w400, y=w403) -> (x+y=w415:dbl)
                n188 = Absolute Value(x=w416) -> (abs(x)=w410:dbl)
                n189 = Divide(x=w415, y=2.0) -> (x/y=w409:dbl)
                n190 = Greater?(x=w412, y=w410) -> (0:w413:bool)
                n191 = case shown="True" w413 {
                  tunnel: w412 -> [_ w466]
                  tunnel: [w464 w466] -> w411
                  tunnel: w410 -> [w464 _]
                  tunnel: w407 -> [_ w465]
                  tunnel: w409 -> [w463 _]
                  tunnel: [w463 w465] -> w408
                  frame False {
                  }
                  frame True {
                  }
                }
                n192 = Increment(x=w421) -> (x+1=w422:dbl)
              }
              frame True {
              }
            }
          }
          n193 = case shown="False" w304 {
            tunnel: w303 -> [w331 _]
            tunnel: [w331 w332] -> w302
            tunnel: w301 -> [_ w332]
            frame False {
            }
            frame True {
            }
          }
          n194 = Subtract(x=w308, y=w302) -> (x-y=w310:dbl)
          n195 = Absolute Value(x=w310) -> (abs(x)=w309:dbl)
          n196 = Add(x=w308, y=w302) -> (x+y=w307:dbl)
          n197 = Greater?(x=w309, y=w314) -> (0:w313:bool)
          n198 = case shown="True" w313 {
            tunnel: [w333 w335] -> w312
            tunnel: w311 -> [w333 _]
            tunnel: w307 -> [_ w334]
            frame False {
            }
            frame True {
              n199 = Divide(x=w334, y=2.0) -> (x/y=w335:dbl)
            }
          }
        }
      }
      "theta final" <- w16
    }
    frame Error {
    }
  }
  "error out" <- w4
  "PositionToReceivePassSkill out" <- w2
